vi "initialize_driver_session.vi"(4 "Supported instruments":string[](array[string]), 5 "Repeated Capabilities":T4[](array[typedef]), 6 "Attributes":T2[](array[typedef]) {"Flags" format="%08b"; "Access" items=["Read Only", "Write Only", "Read/Write"]; "Data Type" items=["Integer 32", "Double", "String", "Boolean", "None", "Integer 64", "RawString"]}, 7 "Range Tables":T3[](array[typedef]) {"Type" items=["Range", "Coerced", "Discrete"]}, 8 "error in":errorcluster caption="error in (no error)", 9 "Option String":string, 10 "Non-VXI sessions list (\"ASRL,SOCKET\")":T1[](array[typedef])=[enum."ASRL", enum."SOCKET"], 11 "VISA resource name":refnum<visa-resource-name>) -> (0 "error out":errorcluster, 2 "Simulation *IDN? response out":string, 3 "VISA resource name out":refnum<visa-resource-name>)   [LabVIEW 2022 SP3, in "hmp4000_rsidr_core.lvlib"]
uses:
  hmp4000_rsidr_core.lvlib
  type_Input_Format_RepCap.ctl
  type_Input_Format_RangeTable.ctl
  type_Input_Format_Attribute.ctl
  type_InterfaceType.ctl
  type_Error_Codes.ctl
  type_Session_Parameter_int32.ctl
  type_Session_Data.ctl
  type_VisaAccessMode.ctl
  type_OPC_Wait_Mode.ctl
  type_Binary_Float_Number_Format.ctl
  type_Binary_Integer_Number_Format.ctl
  _type_Operation_Fgv_Attributes.ctl
  _type_Operation_Fgv_Cache.ctl
  _type_Operation_Fgv_RangeTable.ctl
  type_AdditionalFlag_Bits.ctl
  _type_Operation_Fgv_Session.ctl
  type_Session_Parameter_Boolean.ctl
  Trim Whitespace One-Sided.vi
  Match Regular Expression.xnode
  _type_Operation_Fgv_Debug.ctl
panel:
  # "Attribute Flags:\nbit 0: OPC Wait\nbit 1: No Status Check\nbit 2: Cache only\nbit 3: Hidden"
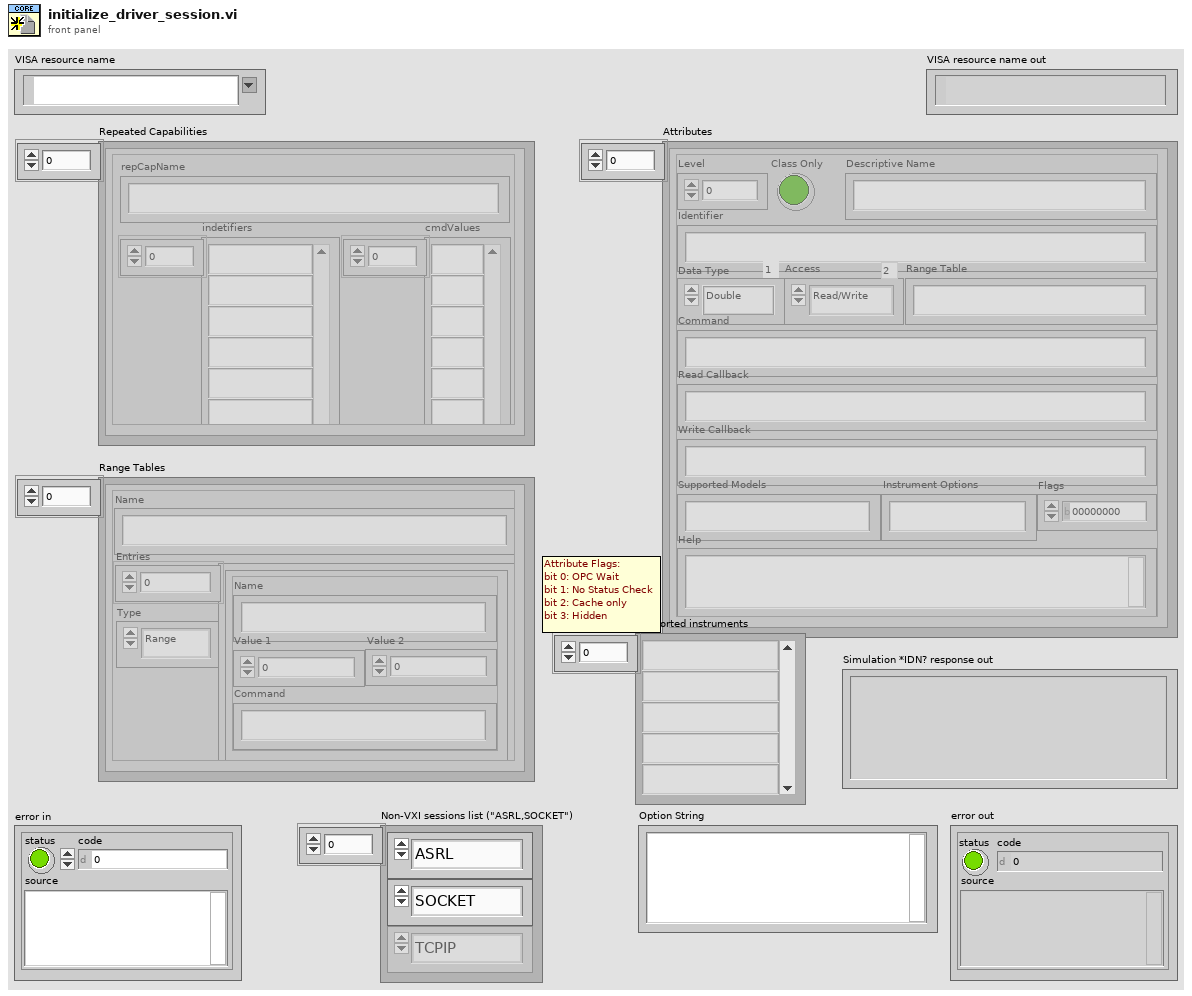
[diagram p1: front panel]
types:
  T1 = typedef "hmp4000_rsidr_core.lvlib/type_InterfaceType.ctl" = enum16{"Unknown", "GPIB", "VXI", "GPIB_VXI", "ASRL", "PXI", "TCPIP", "USB", "SOCKET"}
  T2 = typedef "hmp4000_rsidr_core.lvlib/type_Input_Format_Attribute.ctl" = cluster{"Level":i32, "Class Only":bool, "Identifier":string, "Descriptive Name":string, "Data Type":u16, "Command":string, "Access":u16, "Range Table":string, "Read Callback":string, "Write Callback":string, "Supported Models":string, "Instrument Options":string, "Flags":i32, "Help":string}
  T3 = typedef "hmp4000_rsidr_core.lvlib/type_Input_Format_RangeTable.ctl" = cluster{"Type":u16, "Name":string, "Entries":cluster{"Name":string, "Value 1":dbl, "Value 2":dbl, "Command":string}[]}
  T4 = typedef "hmp4000_rsidr_core.lvlib/type_Input_Format_RepCap.ctl" = cluster{"repCapName":string, "indetifiers":string[], "cmdValues":string[]}
  T5 = typedef "hmp4000_rsidr_core.lvlib/_type_Operation_Fgv_RangeTable.ctl" = enum16{"Initialize", "Check", "Coerce", "Get Command String", "Get Numeric Value", "Get Default Value", "Get Range Table Type"}
  T6 = typedef "hmp4000_rsidr_core.lvlib/_type_Operation_Fgv_Cache.ctl" = enum16{"Initialize", "Get Cached Value", "Set Cached Value", "Clear"}
  T7 = typedef "hmp4000_rsidr_core.lvlib/_type_Operation_Fgv_Attributes.ctl" = enum16{"Initialize", "Get Attribute"}
  T8 = typedef "hmp4000_rsidr_core.lvlib/type_Session_Data.ctl" = cluster{"IDN string":string, "Instrument FW":string, "Instr type":string, "Instr type for err. msg.":string, "Installed Options":string[], "Ignore Error Messages":string, "Logging params":variant, "OPC Timeout":i32, "VISA Timeout":i32, "STB Poll VISA Timeout":i32, "Additional Flags":i32, "Wait Before Read":i32, "Wait Before Write":i32, "Option String Flags":i32, "IO Segment Size":i64, "VISA Access Mode":T9, "Interface Type":T1, "OPC Wait Mode":T10, "Bin Float Number  Format":T11, "Bin Integer Number Format":T12, "Simulate":bool, "VXIcapable":bool, "Duplicate Session":bool, "Add LF to Write":bool, "Logging":bool, "Fast Sweep":bool, "Query Instrument Status":bool, "Check Range":bool, "Check Options":bool}
  T9 = typedef "hmp4000_rsidr_core.lvlib/type_VisaAccessMode.ctl" = u16
  T10 = typedef "hmp4000_rsidr_core.lvlib/type_OPC_Wait_Mode.ctl" = enum16{"STBpolling", "STBpollingSlow", "STBpollingSuperSlow", "ServiceRequest", "OPCquery"}
  T11 = typedef "hmp4000_rsidr_core.lvlib/type_Binary_Float_Number_Format.ctl" = enum16{"Float_4_Bytes_Swapped", "Float_4_Bytes", "Double_8_Bytes_Swapped", "Double_8_Bytes"}
  T12 = typedef "hmp4000_rsidr_core.lvlib/type_Binary_Integer_Number_Format.ctl" = enum16{"Int32_4_Bytes_Swapped", "Int32_4 Bytes", "Int16_2_Bytes_Swapped", "Int16_2_Bytes"}
  T13 = typedef "hmp4000_rsidr_core.lvlib/type_Session_Parameter_int32.ctl" = enum16{"OPC Timeout", "Additional Flags", "Wait Before Write", "Wait Before Read", "Bin Data Chunk Size", "VISA Access Mode", "VISA Timeout", "Bin Float Number Format", "Bin Integer Number Format", "STBpollVISAtimeout", "OPCwaitMode"}
  T14 = typedef "hmp4000_rsidr_core.lvlib/type_Error_Codes.ctl" = enum16{"No_error", "VISA_err_ResourceNotFound", "VISA_err_Timeout", "VISA_warn_MoreDataAvailable", "RS_err_MissingCallback", "RS_err_InvalidAttribute", "RS_err_InvalidValue", "RS_err_UnknownResource", "RS_err_AlreadyInitialized", "RS_err_InstrumentStatus", "RS_err_BadRepCapName", "RS_err_TypesMismatch", "RS_err_ValueNotSupported", "RS_err_InvalidRngTable", "RS_err_IDqueryFail", "RS_err_UnexpResponse", "VISA_warn_ConfigNotLoaded", "RS_err_AttributeNotReadable", "RS_err_AttributeNotWritable", "RS_err_InstrumentType", "RS_err_InstrumentOption", "VISA_err_InvalidSize", "RS_err_ReliabilityIndicator", "VISA_warn_UnknownStatus", "VISA_warn_TermCharRead", "VISA_err_IO_error", "RS_err_FunctionNotSupported", "VISA_warn_QueueEmpty"}
  T15 = typedef "hmp4000_rsidr_core.lvlib/type_AdditionalFlag_Bits.ctl" = enum16{"Send LF after Bin Block", "Junk read with io_clear_buffers.vi", "io_clear_buffers: viClear()", "io_clear_buffers: viFlush()", "<NotUsed1>", "Allow Dbl & Int Bin/Ascii read", "*OPC? in check_instrument_error.vi", "<NotUsed2>", "Smart Enum Matching", "Less Strict RepCaps check", "AssureResponseEndWithLF"}
  T16 = typedef "hmp4000_rsidr_core.lvlib/_type_Operation_Fgv_Session.ctl" = enum16{"Initialize", "GetData", "SetData", "Clear", "GetSessionIx"}
  T17 = typedef "hmp4000_rsidr_core.lvlib/type_Session_Parameter_Boolean.ctl" = enum16{"Simulate", "Query Instr Status", "Check Range", "Check Options", "Add LF to Write", "Duplicate Session", "Fast Sweep", "Logging"}
  T18 = enum16{"Unknown", "GPIB", "VXI", "GPIB_VXI", "ASRL", "PXI", "TCPIP", "USB", "SOCKET"}
  T19 = typedef "hmp4000_rsidr_core.lvlib/_type_Operation_Fgv_Debug.ctl" = enum16{"Reset", "ReadCommand", "SetCommand"}
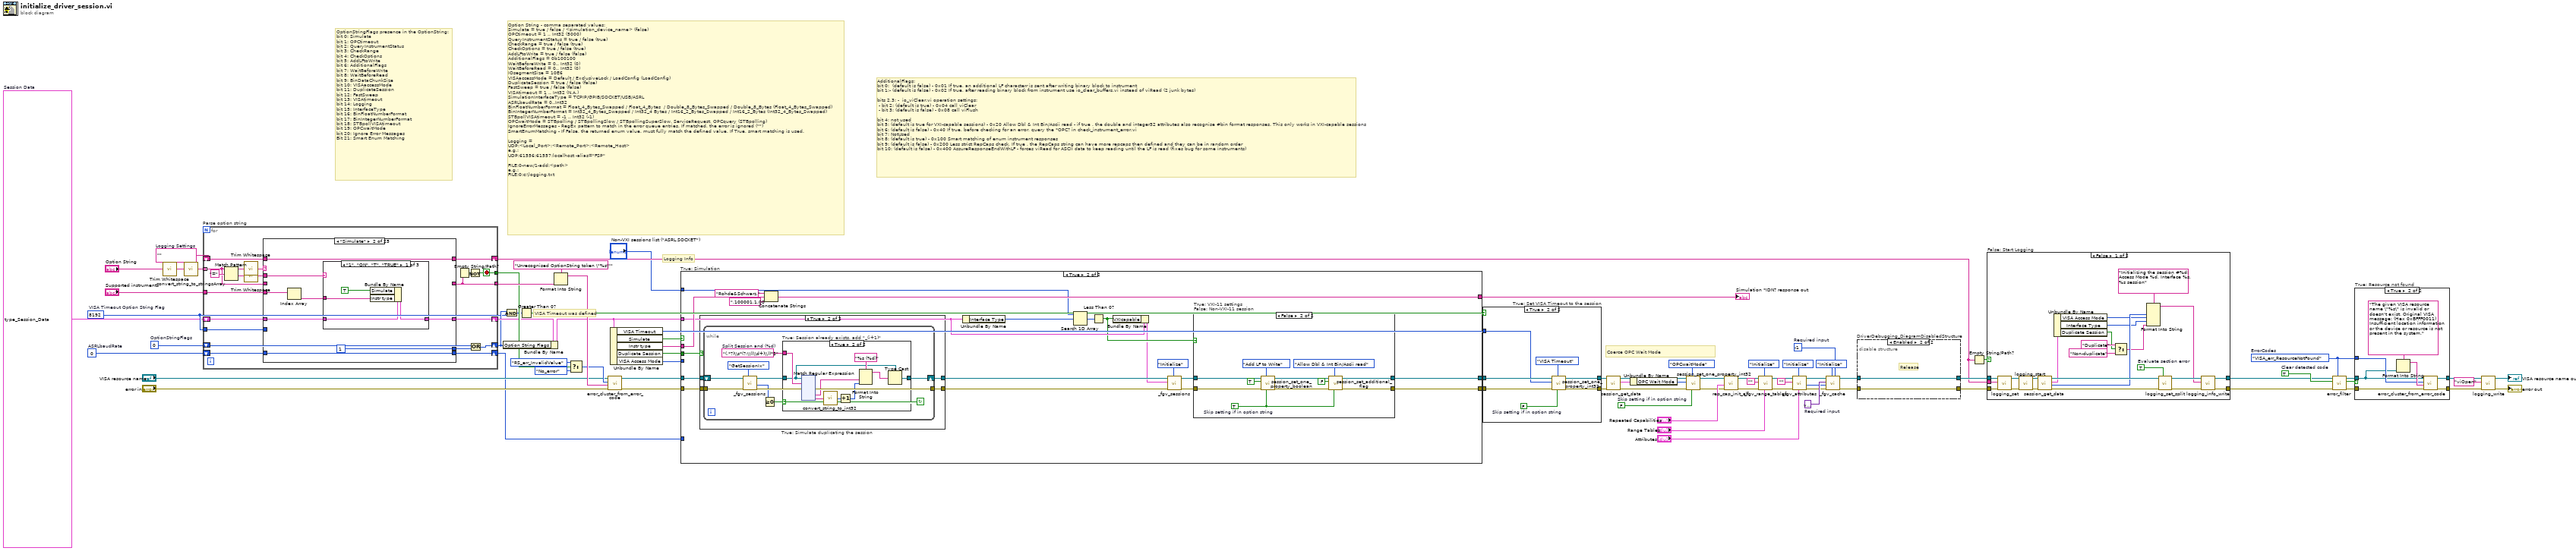
[diagram p0: block diagram]
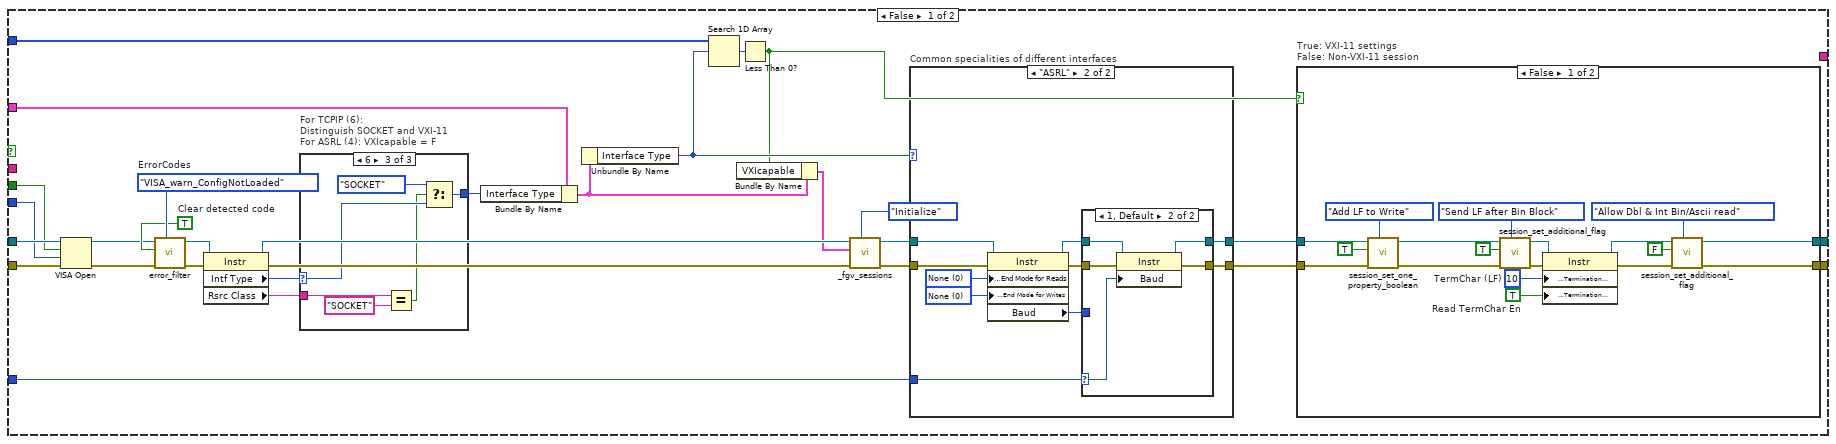
[diagram p3: hidden frame]
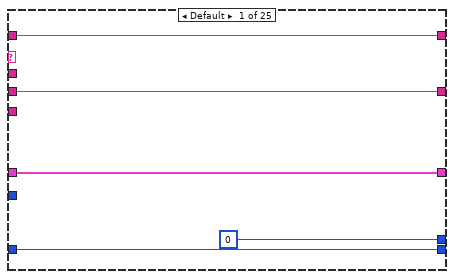
[diagram p14: hidden frame]
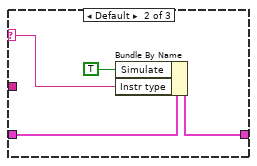
[diagram p15: hidden frame]
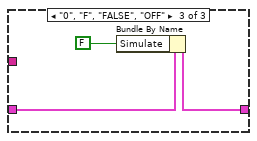
[diagram p16: hidden frame]
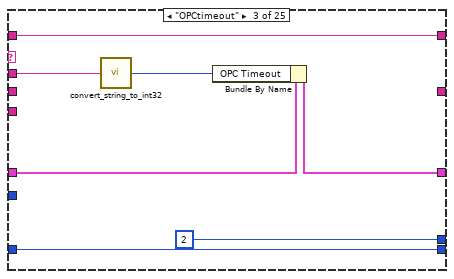
[diagram p17: hidden frame]
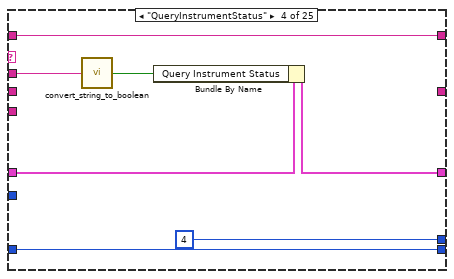
[diagram p18: hidden frame]
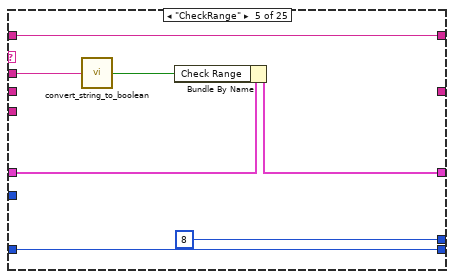
[diagram p19: hidden frame]
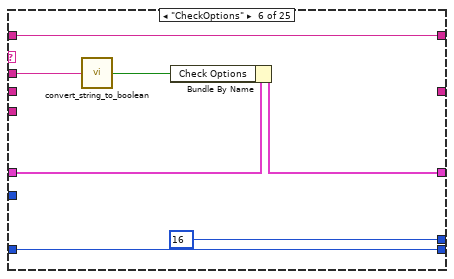
[diagram p20: hidden frame]
diagram:
  w4 = T8 {"IDN string"="", "Instrument FW"="", "Instr type"="", "Instr type for err. msg."="", "Installed Options"=[], "Ignore Error Messages"="", "Logging params"=variant, "OPC Timeout"=10000, "VISA Timeout"=5000, "STB Poll VISA Timeout"=-1, "Additional Flags"=292, "Wait Before Read"=0, "Wait Before Write"=0, "Option String Flags"=0, "IO Segment Size"=10000000, "VISA Access Mode"=4, "Interface Type"=enum."Unknown", "OPC Wait Mode"=enum."STBpolling", "Bin Float Number  Format"=enum."Float_4_Bytes_Swapped", "Bin Integer Number Format"=enum."Int32_4_Bytes_Swapped", "Simulate"=FALSE, "VXIcapable"=FALSE, "Duplicate Session"=FALSE, "Add LF to Write"=FALSE, "Logging"=FALSE, "Fast Sweep"=FALSE, "Query Instrument Status"=TRUE, "Check Range"=TRUE, "Check Options"=TRUE}  # Session Data
  w7 = FALSE  # Skip setting if in option string
  w18 = 0  # ASRLbaudRate
  w31 = 8192  # VISA Timeout Option String Flag
  w37 = 0  # OptionStringFlags
  w57 = type_Error_Codes."VISA_err_ResourceNotFound"  # ErrorCodes
  w59 = TRUE  # Clear detected code
  w66 = ""  # Logging Settings
  w80 = variant  # Required input
  w38 = -1  # Required input
  # "Coerce OPC Wait Mode"
  # "VISA Timeout was defined"
  # "Logging Info"
  # "OptionStringFlags presence in the OptionString:\nbit 0: Simulate\nbit 1: OPCtimeout\nbit 2: QueryInstrumentStatus\nbit 3: CheckRange\nbit 4: CheckOptions\nbit 5: AddLFtoWrite\nbit 6: AdditionalFlags\nbit 7: WaitBeforeWrite\nbit 8: WaitBeforeRead\nbit 9: BinDataChunkSize\nbit 10: VISAaccessMode\nbit 11: DuplicateSession\nbit 12: FastSweep\nbit 13: VISAtimeout\nbit 14: Logging\nbit 15: InterfaceType\nbit 16: BinFloatNumberFormat\nbit 17: BinIntegerNumberFormat\nbit 18: STBpollVISAtimeout\nbit 19: OPCwaitMode\nbit 20: Ignore Error Messages\nBit 21: Smart Enum Matching"
  # "AdditionalFlags:\nbit 0:  (default is false) - 0x01 If true, an additional LF characterr is sent after writing binary block to instrument\nbit 1:- (default is false) - 0x02 If true, after reading binary block from instrument use io_clear_buffers.vi instead of viRead (2 junk bytes)\n\nbits 2,3: -  io_viClear.vi operation settings:\n - bit 2: (default is true) - 0x04 call viClear\n - bit 3: (default is false) - 0x08 call viFlush\n\nbit 4: not used\nbit 5: (default is true for VXI-capable sessions) - 0x20 Allow Dbl & Int Bin/Ascii read - if true , the double and integer32 attributes also recognise #bin format responses. This only works in VXI-capable sessions\nbit 6: (default is false) - 0x40 If true, before checking for an error, query the *OPC? in check_instrument_error.vi\nbit 7: NotUsed\nbit 8: (default is true) - 0x100 Smart matching of enum instrument responses\nbit 9: (default is false) - 0x200 Less strict RepCaps check. If true , the RepCaps string can have more repcaps then defined and they can be in random order\nbit 10: (default is false) - 0x400 AssureResponseEndWithLF - forces viRead for ASCII data to keep reading until the LF is read (fixes bug for some instruments)"
  # "Option String - comma separated values:\nSimulate = true / false / <simulation_device_name> (false)\nOPCtimeout = 1 .. Int32 (5000)\nQueryInstrumentStatus = true / false (true)\nCheckRange = true / false (true)\nCheckOptions = true / false (true)\nAddLFtoWrite = true / false (false)\nAdditionalFlags = 0b100100\nWaitBeforeWrite = 0.. Int32 (0)\nWaitBeforeRead = 0.. Int32 (0)\nIOsegmentSize = 10E6\nVISAaccessMode = Default / ExclusiveLock / LoadConfig (LoadConfig)\nDuplicateSession = true / false (false)\nFastSweep = true / false (false)\nVISAtimeout = 1 .. Int32 (N.A.)\nSimulationInterfaceType = TCPIP/GPIB/SOCKET/USB/ASRL\nASRLbaudRate = 0..Int32\nBinFloatNumberFormat = Float_4_Bytes_Swapped / Float_4_Bytes  / Double_8_Bytes_Swapped / Double_8_Bytes (Float_4_Bytes_Swapped)\nBinIntegerNumberFormat = Int32_4_Bytes_Swapped / Int32_4 Bytes / Int16_2_Bytes_Swapped / Int16_2_Bytes (Int32_4_Bytes_Swapped)\nSTBpollVISAtimeout = -1 .. Int32 (-1)\nOPCwaitMode = STBpolling / STBpollingSlow / STBpollingSuperSlow, ServiceRequest, OPCquery (STBpolling)\nIgnoreErrorMessages - RegEx pattern to match in the error queue entries. If matched, the error is ignored (\"\")\nSmartEnumMatching - If False, the returned enum value. must fully match the defined value. If True, smart matching is used.\n\nLogging =\nUDP:<Local_Port>:<Remote_Port>:<Remote_Host>\ne.g.:\nUDP:61556:61557:localhost -alias=\"FSP\"\n\nFILE:0-new/1-add:<path>\ne.g.:\nFILE:0:c:\\logging.txt"
  n1 = call "Trim Whitespace.vi"("string"="Option String") -> ("trimmed string"=w6:string)  [unwired: 1 in]
  n2 = call "convert_string_to_stringsArray.vi"("String in"=w6) -> ("string array out"=w70:string[])  [unwired: 3 in, 1 out]
  n3 = for "Parse option string" {
    tunnel: w70 -> [w94] mode=indexing
    shift-right: [w96] -> w33
    shift-left: w4 -> [w97]
    tunnel: "Supported instruments" -> [w92]
    shift-right: [w90] -> w64
    shift-left: w66 -> [w91]
    tunnel: [w88] -> w44
    tunnel: [w87] -> w43
    shift-right: [w85] -> w32
    shift-left: w37 -> [w86]
    tunnel: w31 -> [w83]
    shift-right: [w81] -> w17
    shift-left: w18 -> [w82]
    stop <- w87 stop-if-true
    n4 = Match Pattern(string=w94, regular expression="=") -> (before substring=w99:string, after substring=w98:string)  [unwired: 1 in, 2 out]
    n5 = call "Trim Whitespace.vi"("string"=w99) -> ("trimmed string"=w95:string)  [unwired: 1 in]
    n6 = call "Trim Whitespace.vi"("string"=w98) -> ("trimmed string"=w93:string)  [unwired: 1 in]
    n7 = case shown="\"Simulate\"" w95 {
      tunnel: w97 -> [w105 w107 w131 w133 w140 w152 w154 w166 w173 w183 w190 w198 w200 w214 w221 w228 w235 w241 w244 w260 w275 w291 w297 w314 w324]
      tunnel: [w105 w106 w130 w132 w139 w146 w153 w165 w174 w182 w189 w197 w199 w213 w220 w227 w235 w241 w243 w259 w274 w290 w296 w313 w325] -> w96
      tunnel: w94 -> [w103 _ _ _ _ _ _ _ _ _ _ _ w205 _ _ _ _ _ w249 w265 w280 _ w302 _ _]
      tunnel: w93 -> [_ w109 w128 w137 w144 w150 w158 w163 w170 w180 w187 w195 w207 w218 w225 w232 w237 w242 w251 w267 w282 w293 w304 w312 w321]
      tunnel: w92 -> [_ w113 _ _ _ _ _ _ _ _ _ _ _ _ _ _ _ _ _ _ _ _ _ _ _]
      tunnel: w91 -> [w104 w112 w129 w138 w145 w151 w159 w164 w176 w181 w188 w196 w206 w219 w226 w233 w238 _ w250 w266 w281 w289 w303 w317 w327]
      tunnel: [w104 w112 w129 w138 w145 w151 w159 w164 w176 w181 w188 w196 w206 w219 w226 w233 w238 w242 w250 w266 w281 w289 w303 w317 w327] -> w90
      tunnel: [w103 _ _ _ _ _ _ _ _ _ _ _ w204 _ _ _ _ _ w248 w264 w279 _ w301 _ _] -> w88
      tunnel: [0 ("y") 1 ("y") 2 ("y") 4 ("y") 8 ("y") 16 ("y") 32 ("y") 64 ("y") 64 ("y") 128 ("y") 256 ("y") 512 ("y") 1024 ("y") 2048 ("y") 4096 ("y") w230 w234 16384 ("y") 32768 ("y") 65536 ("y") 131072 ("y") 262144 ("y") 524288 ("y") 1048576 ("y") 64 ("y")] -> w84
      tunnel: w83 -> [_ _ _ _ _ _ _ _ _ _ _ _ _ _ _ w230 _ _ _ _ _ _ _ _ _]
      tunnel: w82 -> [w101 w110 w125 w134 w141 w147 w155 w160 w175 w177 w184 w192 w201 w215 w222 w229 _ w239 w245 w261 w276 w294 w298 w315 w326]
      tunnel: [w101 w110 w125 w134 w141 w147 w155 w160 w175 w177 w184 w192 w201 w215 w222 w229 w236 w239 w245 w261 w276 w294 w298 w315 w326] -> w81
      frame Default {
      }
      frame "Simulate" {
        n8 = Index Array(array=w113) -> (element=w108:string)  [unwired: 1 in]
        n9 = case shown="\"1\", \"ON\", \"T\", \"TRUE\"" w109 {
          selector: w109 -> [_ w118 _]
          tunnel: w107 -> [w117 w121 w124]
          tunnel: [w116 w120 w123] -> w106
          tunnel: w108 -> [w115 _ _]
          frame "1", "ON", "T", "TRUE" {
            n10 = Bundle By Name(cluster=w117, "Simulate"=TRUE ("Simulation"), "Instr type"=w115) -> (w116:T8)
          }
          frame Default {
            n11 = Bundle By Name(cluster=w121, "Simulate"=TRUE ("Simulation"), "Instr type"=w118) -> (w120:T8)
          }
          frame "0", "F", "FALSE", "OFF" {
            n12 = Bundle By Name(cluster=w124, "Simulate"=FALSE ("Simulation")) -> (w123:T8)
          }
        }
      }
      frame "OPCtimeout" {
        n13 = call "convert_string_to_int32.vi"("String in"=w128) -> ("int32 value out"=w127:i32)  [unwired: 4 in]
        n14 = Bundle By Name(cluster=w131, "OPC Timeout"=w127) -> (w130:T8)
      }
      frame "QueryInstrumentStatus" {
        n15 = call "convert_string_to_boolean.vi"("String in"=w137) -> ("boolean value out"=w136:bool)  [unwired: 4 in]
        n16 = Bundle By Name(cluster=w133, "Query Instrument Status"=w136) -> (w132:T8)
      }
      frame "CheckRange" {
        n17 = call "convert_string_to_boolean.vi"("String in"=w144) -> ("boolean value out"=w143:bool)  [unwired: 4 in]
        n18 = Bundle By Name(cluster=w140, "Check Range"=w143) -> (w139:T8)
      }
      frame "CheckOptions" {
        n19 = call "convert_string_to_boolean.vi"("String in"=w150) -> ("boolean value out"=w149:bool)  [unwired: 4 in]
        n20 = Bundle By Name(cluster=w152, "Check Options"=w149) -> (w146:T8)
      }
      frame "AddLFtoWrite" {
        n21 = call "convert_string_to_boolean.vi"("String in"=w158) -> ("boolean value out"=w157:bool)  [unwired: 4 in]
        n22 = Bundle By Name(cluster=w154, "Add LF to Write"=w157) -> (w153:T8)
      }
      frame "AdditionalFlags" {
        n23 = call "convert_string_to_int32.vi"("String in"=w163) -> ("int32 value out"=w162:i32)  [unwired: 4 in]
        n24 = Bundle By Name(cluster=w166, "Additional Flags"=w162) -> (w165:T8)
      }
      frame "AssureResponseEndWithLF" {
        n25 = Unbundle By Name(w173) -> ("Additional Flags"=w172:i32)
        n26 = call "convert_string_to_boolean.vi"("String in"=w170) -> ("boolean value out"=w169:bool)  [unwired: 4 in]
        n27 = call "_session_set_additionalFlag_value.vi"("New value in"=w169, "AdditionalFlag bit"=type_AdditionalFlag_Bits."AssureResponseEndWithLF", "Additional Flags in"=w172) -> ("Additional Flags out"=w168:i32)  [unwired: 1 in, 1 out]
        n28 = Bundle By Name(cluster=w173, "Additional Flags"=w168) -> (w174:T8)
      }
      frame "WaitBeforeWrite" {
        n29 = call "convert_string_to_int32.vi"("String in"=w180) -> ("int32 value out"=w179:i32)  [unwired: 4 in]
        n30 = Bundle By Name(cluster=w183, "Wait Before Write"=w179) -> (w182:T8)
      }
      frame "WaitBeforeRead" {
        n31 = call "convert_string_to_int32.vi"("String in"=w187) -> ("int32 value out"=w186:i32)  [unwired: 4 in]
        n32 = Bundle By Name(cluster=w190, "Wait Before Read"=w186) -> (w189:T8)
      }
      frame "IOsegmentSize" {
        n33 = call "convert_string_to_int32.vi"("String in"=w195) -> ("int32 value out"=w194:i32)  [unwired: 4 in]
        n34 = To Quad Integer(1:w194) -> (0:w191:i64)
        n35 = Bundle By Name(cluster=w198, "IO Segment Size"=w191) -> (w197:T8)
      }
      frame "VISAaccessMode" {
        n36 = case shown="\"LoadConfig\"" w207 {
          tunnel: w205 -> [_ w210 _ _]
          tunnel: [_ w210 _ _] -> w204
          tunnel: [w208 w209 w211 w212] -> w203
          frame "Default" {
            w208 = T9 0 items=["VISA Defaults"=0, "Exclusive Lock"=1, "Load Settings"=4]  # VISA Access Mode
          }
          frame Default {
            w209 = T9 4 items=["VISA Defaults"=0, "Exclusive Lock"=1, "Load Settings"=4]  # VISA Access Mode
          }
          frame "ExclusiveLock" {
            w211 = T9 1 items=["VISA Defaults"=0, "Exclusive Lock"=1, "Load Settings"=4]  # VISA Access Mode
          }
          frame "LoadConfig" {
            w212 = T9 4 items=["VISA Defaults"=0, "Exclusive Lock"=1, "Load Settings"=4]  # VISA Access Mode
          }
        }
        n37 = Bundle By Name(cluster=w200, "VISA Access Mode"=w203) -> (w199:T8)
      }
      frame "DuplicateSession" {
        n38 = call "convert_string_to_boolean.vi"("String in"=w218) -> ("boolean value out"=w217:bool)  [unwired: 4 in]
        n39 = Bundle By Name(cluster=w214, "Duplicate Session"=w217) -> (w213:T8)
      }
      frame "FastSweep" {
        n40 = call "convert_string_to_boolean.vi"("String in"=w225) -> ("boolean value out"=w224:bool)  [unwired: 4 in]
        n41 = Bundle By Name(cluster=w221, "Fast Sweep"=w224) -> (w220:T8)
      }
      frame "VISAtimeout" {
        n42 = call "convert_string_to_int32.vi"("String in"=w232) -> ("int32 value out"=w231:i32)  [unwired: 4 in]
        n43 = Bundle By Name(cluster=w228, "VISA Timeout"=w231) -> (w227:T8)
      }
      frame "ASRLbaudRate" {
        w234 = 0  # OptionStringFlags
        n44 = call "convert_string_to_int32.vi"("String in"=w237) -> ("int32 value out"=w236:i32)  [unwired: 4 in]
      }
      frame "Logging" {
      }
      frame "SimulationInterfaceType" {
        n45 = case shown="\"ASRL\"" w251 {
          tunnel: w249 -> [w253 _ _ _ _ _]
          tunnel: [w253 _ _ _ _ _] -> w248
          tunnel: [type_InterfaceType."TCPIP" ("Interface Type") type_InterfaceType."TCPIP" ("Interface Type") type_InterfaceType."GPIB" ("Interface Type") type_InterfaceType."SOCKET" ("Interface Type") type_InterfaceType."USB" ("Interface Type") type_InterfaceType."ASRL" ("Interface Type")] -> w247
          frame Default {
          }
          frame "TCPIP" {
          }
          frame "GPIB" {
          }
          frame "SOCKET" {
          }
          frame "USB" {
          }
          frame "ASRL" {
          }
        }
        n46 = Bundle By Name(cluster=w244, "Interface Type"=w247) -> (w243:T8)
      }
      frame "BinFloatNumberFormat" {
        n47 = case shown="\"Double_8_Bytes_Swapped\"" w267 {
          tunnel: w265 -> [w269 _ _ _ _]
          tunnel: [w269 _ _ _ _] -> w264
          tunnel: [w268 w270 w271 w272 w273] -> w263
          frame Default {
            w268 = type_Binary_Float_Number_Format."Float_4_Bytes_Swapped"  # Bin Number Format
          }
          frame "Float_4_Bytes_Swapped" {
            w270 = type_Binary_Float_Number_Format."Float_4_Bytes_Swapped"  # Bin Float Number Format
          }
          frame "Float_4_Bytes" {
            w271 = type_Binary_Float_Number_Format."Float_4_Bytes"  # Bin Float Number Format
          }
          frame "Double_8_Bytes_Swapped" {
            w272 = type_Binary_Float_Number_Format."Double_8_Bytes_Swapped"  # Bin Float Number Format
          }
          frame "Double_8_Bytes" {
            w273 = type_Binary_Float_Number_Format."Double_8_Bytes"  # Bin Float Number Format
          }
        }
        n48 = Bundle By Name(cluster=w260, "Bin Float Number  Format"=w263) -> (w259:T8)
      }
      frame "BinIntegerNumberFormat" {
        n49 = case shown="\"Int16_2_Bytes_Swapped\"" w282 {
          tunnel: w280 -> [w284 _ _ _ _]
          tunnel: [w284 _ _ _ _] -> w279
          tunnel: [w283 w285 w286 w287 w288] -> w278
          frame Default {
            w283 = type_Binary_Integer_Number_Format."Int32_4_Bytes_Swapped"  # Bin Integer Number Format
          }
          frame "Int32_4_Bytes_Swapped" {
            w285 = type_Binary_Integer_Number_Format."Int32_4_Bytes_Swapped"  # Bin Integer Number Format
          }
          frame "Int32_4_Bytes" {
            w286 = type_Binary_Integer_Number_Format."Int32_4 Bytes"  # Bin Integer Number Format
          }
          frame "Int16_2_Bytes_Swapped" {
            w287 = type_Binary_Integer_Number_Format."Int16_2_Bytes_Swapped"  # Bin Integer Number Format
          }
          frame "Int16_2_Bytes" {
            w288 = type_Binary_Integer_Number_Format."Int16_2_Bytes"  # Bin Integer Number Format
          }
        }
        n50 = Bundle By Name(cluster=w275, "Bin Integer Number Format"=w278) -> (w274:T8)
      }
      frame "STBpollVISAtimeout" {
        n51 = call "convert_string_to_int32.vi"("String in"=w293) -> ("int32 value out"=w292:i32)  [unwired: 4 in]
        n52 = Bundle By Name(cluster=w291, "STB Poll VISA Timeout"=w292) -> (w290:T8)
      }
      frame "OPCwaitMode" {
        n53 = case shown="\"ServiceRequest\"" w304 {
          tunnel: w302 -> [_ _ _ _ _ w310]
          tunnel: [_ _ _ _ _ w310] -> w301
          tunnel: [w305 w306 w307 w308 w309 w311] -> w300
          frame "STBpolling" {
            w305 = type_OPC_Wait_Mode."STBpolling"  # OPC Wait Mode
          }
          frame "STBpollingSlow" {
            w306 = type_OPC_Wait_Mode."STBpollingSlow"  # OPC Wait Mode
          }
          frame "STBpollingSuperSlow" {
            w307 = type_OPC_Wait_Mode."STBpollingSuperSlow"  # OPC Wait Mode
          }
          frame "ServiceRequest" {
            w308 = type_OPC_Wait_Mode."ServiceRequest"  # OPC Wait Mode
          }
          frame "OPCquery" {
            w309 = type_OPC_Wait_Mode."OPCquery"  # OPC Wait Mode
          }
          frame Default {
            w311 = type_OPC_Wait_Mode."STBpolling"  # OPC Wait Mode
          }
        }
        n54 = Bundle By Name(cluster=w297, "OPC Wait Mode"=w300) -> (w296:T8)
      }
      frame "IgnoreErrorMessages" {
        n55 = Bundle By Name(cluster=w314, "Ignore Error Messages"=w312) -> (w313:T8)
      }
      frame "SmartEnumMatching" {
        n56 = Unbundle By Name(w324) -> ("Additional Flags"=w323:i32)
        n57 = call "convert_string_to_boolean.vi"("String in"=w321) -> ("boolean value out"=w320:bool)  [unwired: 4 in]
        n58 = call "_session_set_additionalFlag_value.vi"("New value in"=w320, "AdditionalFlag bit"=type_AdditionalFlag_Bits."Smart Enum Matching", "Additional Flags in"=w323) -> ("Additional Flags out"=w319:i32)  [unwired: 1 in, 1 out]
        n59 = Bundle By Name(cluster=w324, "Additional Flags"=w319) -> (w325:T8)
      }
    }
    n60 = Empty String/Path?(string/path=w88) -> (empty?=w89:bool)
    n61 = Not(x=w89) -> (.not. x?=w87:bool)
    n62 = Or(x=w86, y=w84) -> (x .or. y?=w85:i32)
  }
  n63 = Bundle By Name(cluster=w33, "Option String Flags"=w32) -> (w36:T8)
  n64 = And(x=w32, y=w31) -> (x .and. y?=w30:i32)
  n65 = Greater Than 0?(x=w30) -> (x > 0?=w29:bool)
  n66 = Format Into String(format string="Unrecognised OptionString token \"%s\"", w44) -> (resulting string=w46:string)  [unwired: 2 in, 1 out]
  n67 = Select(t=type_Error_Codes."RS_err_InvalidValue" ("Error Enum in"), s=w43, f=type_Error_Codes."No_error" ("Error Enum in")) -> (s? t:f=w40:T14)
  n68 = call "error_cluster_from_error_code.vi"("error in"="error in", "Error Message (\"\")"=w46, "Error Enum in"=w40, "VISA resource name"="VISA resource name") -> ("error out"=w25:errorcluster, "VISA resource name out"=w24:refnum<visa-resource-name>)  [unwired: 6 in]
  n69 = Unbundle By Name(w36) -> ("VISA Timeout"=w28:i32, "Simulate"=w56:bool, "Instr type"=w58:string, "Duplicate Session"=w23:bool, "VISA Access Mode"=w22:T9)
  n70 = case "True: Simulation" shown="True" w56 {
    tunnel: w24 -> [w356 w421]
    tunnel: w25 -> [w357 w420]
    tunnel: [w336 w414] -> w35
    tunnel: [w335 w413] -> w34
    tunnel: w58 -> [_ w419]
    tunnel: [_ w423] -> w55
    tunnel: w36 -> [w346 w412]
    tunnel: w23 -> [w349 w422]
    tunnel: w22 -> [w348 _]
    tunnel: w17 -> [w339 _]
    tunnel: "Non-VXI sessions list (\"ASRL,SOCKET\")" -> [w333 w410]
    frame False {
      w350 = TRUE  # Clear detected code
      w353 = type_Error_Codes."VISA_warn_ConfigNotLoaded"  # ErrorCodes
      n71 = VISA Open ("Open instrument")(duplicate session (F)=w349, access mode=w348, error in (no error)=w357, VISA resource name=w356) -> (VISA resource name=w345:refnum<visa-resource-name>, error out=w344:errorcluster)  [unwired: 1 in]
      n72 = call "error_filter.vi"("Error Enum in"=w353, "error in"=w344, "Clear detected code (F)"=w350, "VISA resource name"=w345) -> ("error out"=w352:errorcluster, "VISA resource name out"=w351:refnum<visa-resource-name>)  [unwired: 5 in, 1 out]
      n73 = property on="Property Node" class="Instr"(reference=w351, error in=w352) -> (reference out=w342:refnum<visa-resource-name>, error out=w343:errorcluster, "Intf Type"=w355:u16, "Rsrc Class"=w354:string)
      n74 = case "For TCPIP (6):\nDistinguish SOCKET and VXI-11\nFor ASRL (4): VXIcapable = F" shown="6" w355 {
        selector: w355 -> [w397 w398 w402]
        tunnel: w354 -> [_ _ w404]
        tunnel: [w397 w398 w401] -> w347
        frame Default {
        }
        frame 4 {
        }
        frame 6 {
          n75 = Equal?(x=w404, y="SOCKET") -> (x = y?=w399:bool)
          n76 = Select(t=T18."SOCKET" ("Interface Type"), s=w399, f=w402) -> (s? t:f=w401:u16)
        }
      }
      n77 = Bundle By Name(cluster=w346, "Interface Type"=w347) -> (w330:T8)
      n78 = Unbundle By Name(w330) -> ("Interface Type"=w332:T1)
      n79 = Search 1D Array(1D array=w333, element=w332) -> (index of element=w334:i32)  [unwired: 1 in]
      n80 = Less Than 0?(x=w334) -> (x < 0?=w329:bool)
      n81 = Bundle By Name(cluster=w330, "VXIcapable"=w329) -> (w331:T8)
      n82 = call "_fgv_sessions.vi"("Operation"=_type_Operation_Fgv_Session."Initialize", "error in"=w343, "Session User Data in (None)"=w331, "VISA resource name"=w342) -> ("error out"=w341:errorcluster, "VISA resource name out"=w340:refnum<visa-resource-name>)  [unwired: 4 in, 2 out]
      n83 = case "Common specialities of different interfaces" shown="\"ASRL\"" w332 {
        tunnel: w341 -> [w378 w382]
        tunnel: w340 -> [w379 w381]
        tunnel: [w378 w384] -> w338
        tunnel: [w379 w383] -> w337
        tunnel: w339 -> [_ w387]
        frame Default {
        }
        frame "ASRL" {
          w388 = u16 0 items=["None", "Last Bit", "TermChar", "Break"] ("Serial Settings:End Mode for Writes")
          w389 = u16 0 items=["None", "Last Bit", "TermChar"] ("Serial Settings:End Mode for Reads")
          n84 = property on="Property Node" class="Instr"(reference=w381, error in=w382, "Serial Settings:End Mode for Reads"=w389, "Serial Settings:End Mode for Writes"=w388) -> (reference out=w385:refnum<visa-resource-name>, error out=w386:errorcluster, "Baud"=w380:u32)
          n85 = case shown="1, Default" w387 {
            selector: w387 -> [_ w392]
            tunnel: w386 -> [w390 w396]
            tunnel: w385 -> [w391 w393]
            tunnel: [w390 w395] -> w384
            tunnel: [w391 w394] -> w383
            tunnel: w380 -> [_ _]
            frame 0 {
            }
            frame 1, Default {
              n86 = property on="Property Node" class="Instr"(reference=w393, error in=w396, "Baud"=w392) -> (reference out=w394:refnum<visa-resource-name>, error out=w395:errorcluster)
            }
          }
        }
      }
      n87 = case "True: VXI-11 settings\nFalse: Non-VXI-11 session" shown="False" w329 {
        tunnel: w338 -> [w372 w376]
        tunnel: w337 -> [w373 w377]
        tunnel: [w361 w376] -> w336
        tunnel: [w360 w377] -> w335
        frame False {
          w374 = u8 10  # TermChar (LF)
          w375 = TRUE  # Read TermChar En
          n88 = call "session_set_one_property_boolean.vi"("Session Parameter Boolean"=type_Session_Parameter_Boolean."Add LF to Write" ("Session Parameter boolean"), "error in"=w372, "Boolean value in"=TRUE ("boolean value in"), "VISA resource name"=w373) -> ("error out"=w369:errorcluster, "VISA resource name out"=w370:refnum<visa-resource-name>)  [unwired: 5 in, 1 out]
          n89 = call "session_set_additional_flag.vi"("AdditionalFlag Bit"=type_AdditionalFlag_Bits."Send LF after Bin Block" ("AdditionalFlag bit"), "error in"=w369, "New value in"=TRUE, "VISA resource name"=w370) -> ("error out"=w367:errorcluster, "VISA resource name out"=w368:refnum<visa-resource-name>)  [unwired: 5 in, 1 out]
          n90 = property on="Property Node" class="Instr"(reference=w368, error in=w367, "Message Based Settings:Termination Character"=w374, "Message Based Settings:Termination Character Enable"=w375) -> (reference out=w359:refnum<visa-resource-name>, error out=w362:errorcluster)
          n91 = call "session_set_additional_flag.vi"("AdditionalFlag Bit"=type_AdditionalFlag_Bits."Allow Dbl & Int Bin/Ascii read" ("AdditionalFlag bit"), "error in"=w362, "New value in"=FALSE, "VISA resource name"=w359) -> ("error out"=w361:errorcluster, "VISA resource name out"=w360:refnum<visa-resource-name>)  [unwired: 5 in, 1 out]
        }
        frame True {
        }
      }
    }
    frame True {
      n92 = case "True: Simulate duplicating the session" shown="True" w422 {
        tunnel: w421 -> [w439 w441]
        tunnel: [w439 w440] -> w417
        tunnel: w420 -> [w438 w443]
        tunnel: [w438 w442] -> w418
        frame False {
        }
        frame True {
          n93 = while {
            tunnel: w443 -> [w452]
            tunnel: [w451] -> w442
            shift-right: [w446] -> w440
            shift-left: w441 -> [w450]
            stop <- w445 continue-if-true
            w447 = "(.*?)\\s*(?:\\((\\d+)\\))*$"  # Split Session and (%d)
            n94 = call "_fgv_sessions.vi"("Operation"=_type_Operation_Fgv_Session."GetSessionIx", "error in"=w452, "VISA resource name"=w450) -> ("error out"=w451:errorcluster, "Session Ix out"=w449:i32, "VISA resource name out"=w448:refnum<visa-resource-name>)  [unwired: 5 in, 1 out]
            n95 = Greater Or Equal To 0?(x=w449) -> (x >= 0?=w445:bool)
            n96 = case "True: Session already exists, add \"_(i+1)\"" shown="True" w445 {
              tunnel: w448 -> [w453 w454]
              tunnel: w447 -> [_ w462]
              tunnel: [w453 w455] -> w446
              frame False {
              }
              frame True {
                n97 = xnode "Match Regular Expression"("input string"=w454, "regular expression"=w462) -> ("submatch 1"=w458:string, "submatch 2"=w461:string)  [unwired: 4 in, 5 out]
                n98 = call "convert_string_to_int32.vi"("String in"=w461) -> ("int32 value out"=w460:i32)  [unwired: 4 in]
                n99 = Increment(x=w460) -> (x+1=w457:i32)
                n100 = Format Into String(format string="%s (%d)", w458, w457) -> (resulting string=w456:string)  [unwired: 2 in, 1 out]
                n101 = Type Cast(type=w454, x=w456) -> (*(type *) &x=w455:refnum<visa-resource-name>)
              }
            }
          }
        }
      }
      n102 = Concatenate Strings("Rohde&Schwarz," ("read buffer"), w419, ",100001,1.00" ("string")) -> (w423:string)
      n103 = Unbundle By Name(w412) -> ("Interface Type"=w411:T1)
      n104 = Search 1D Array(1D array=w410, element=w411) -> (index of element=w409:i32)  [unwired: 1 in]
      n105 = Less Than 0?(x=w409) -> (x < 0?=w408:bool)
      n106 = Bundle By Name(cluster=w412, "VXIcapable"=w408) -> (w407:T8)
      n107 = call "_fgv_sessions.vi"("Operation"=_type_Operation_Fgv_Session."Initialize", "error in"=w418, "Session User Data in (None)"=w407, "VISA resource name"=w417) -> ("error out"=w416:errorcluster, "VISA resource name out"=w415:refnum<visa-resource-name>)  [unwired: 4 in, 2 out]
      n108 = case "True: VXI-11 settings\nFalse: Non-VXI-11 session" shown="False" w408 {
        tunnel: w416 -> [w425 w436]
        tunnel: w415 -> [w426 w435]
        tunnel: [w425 w431] -> w414
        tunnel: [w426 w430] -> w413
        frame True {
        }
        frame False {
          w427 = TRUE  # Skip setting if in option string
          n109 = call "session_set_one_property_boolean.vi"("Skip setting if in Options string (F)"=w427, "Session Parameter Boolean"=type_Session_Parameter_Boolean."Add LF to Write" ("Session Parameter boolean"), "error in"=w436, "Boolean value in"=TRUE ("boolean value in"), "VISA resource name"=w435) -> ("error out"=w433:errorcluster, "VISA resource name out"=w432:refnum<visa-resource-name>)  [unwired: 4 in, 1 out]
          n110 = call "session_set_additional_flag.vi"("Skip setting if in Options string (F)"=w427, "AdditionalFlag Bit"=type_AdditionalFlag_Bits."Allow Dbl & Int Bin/Ascii read" ("AdditionalFlag bit"), "error in"=w433, "New value in"=FALSE, "VISA resource name"=w432) -> ("error out"=w431:errorcluster, "VISA resource name out"=w430:refnum<visa-resource-name>)  [unwired: 4 in, 1 out]
        }
      }
    }
  }
  "Simulation *IDN? response out" <- w55
  n111 = case "True: Set VISA Timeout to the session" shown="True" w29 {
    tunnel: w35 -> [w583 w591]
    tunnel: w34 -> [w584 w590]
    tunnel: [w583 w589] -> w13
    tunnel: [w584 w588] -> w12
    tunnel: w28 -> [_ w587]
    frame False {
    }
    frame True {
      w585 = FALSE  # Skip setting if in option string
      n112 = call "session_set_one_property_int32.vi"("Skip setting if in Options string (F)"=w585, "Session Parameter Integer"=type_Session_Parameter_int32."VISA Timeout" ("Session Parameter to set"), "error in"=w591, "Int32 value in"=w587, "VISA resource name"=w590) -> ("error out"=w589:errorcluster, "VISA resource name out"=w588:refnum<visa-resource-name>)  [unwired: 4 in, 1 out]
    }
  }
  n113 = call "session_get_data.vi"("error in"=w13, "VISA resource name"=w12) -> ("error out"=w11:errorcluster, "Session User Data out"=w9:T8, "VISA resource name out"=w10:refnum<visa-resource-name>)  [unwired: 6 in, 1 out]
  n114 = Unbundle By Name(w9) -> ("OPC Wait Mode"=w8:T10)
  n115 = call "session_set_one_property_int32.vi"("Skip setting if in Options string (F)"=w7, "Session Parameter Integer"=type_Session_Parameter_int32."OPCwaitMode" ("Session Parameter to set"), "error in"=w11, "Int32 value in"=w8, "VISA resource name"=w10) -> ("error out"=w15:errorcluster, "VISA resource name out"=w14:refnum<visa-resource-name>)  [unwired: 4 in, 1 out]
  n116 = call "rep_cap_init_all.vi"("error in"=w15, "Repeated Capabilities"="Repeated Capabilities", "VISA resource name"=w14) -> ("error out"=w63:errorcluster, "VISA resource name out"=w21:refnum<visa-resource-name>)  [unwired: 7 in]
  n117 = call "_fgv_range_tables.vi"("Range Tables (empty)"="Range Tables", "Operation"=_type_Operation_Fgv_RangeTable."Initialize", "error in"=w63, "Range Table ID in"="" ("Empty String Constant"), "VISA resource name"=w21) -> ("error out"=w77:errorcluster, "VISA resource name out"=w19:refnum<visa-resource-name>)  [unwired: 2 in, 3 out]
  n118 = call "_fgv_attributes.vi"("Attributes (empty)"="Attributes", "Operation"=_type_Operation_Fgv_Attributes."Initialize", "error in"=w77, "Attribute ID in"="" ("Empty String Constant"), "VISA resource name"=w19) -> ("error out"=w76:errorcluster, "Count Out"=w39:i32, "VISA resource name out"=w20:refnum<visa-resource-name>)  [unwired: 3 in, 1 out]
  n119 = call "_fgv_cache.vi"("Index in"=w38, "Operation"=_type_Operation_Fgv_Cache."Initialize", "error in"=w76, "Initialization Count (0)"=w39, "Value in"=w80, "VISA resource name"=w20) -> ("error out"=w73:errorcluster, "VISA resource name out"=w72:refnum<visa-resource-name>)  [unwired: 3 in, 1 out]
  n120 = disable-structure "DriverDebugging_DiagramDisabledStructure" shown="Enabled" {
    disable-tunnel: w73 -> [w597 w598]
    disable-tunnel: [w595 w598] -> w68
    disable-tunnel: w72 -> [w596 w599]
    disable-tunnel: [w594 w599] -> w67
    frame Disabled {
      # "Debug"
      n121 = call "_fgv_debug.vi"("Operation"=_type_Operation_Fgv_Debug."Reset", "error in"=w597, "Command in"="" ("Empty String Constant"), "VISA resource name"=w596) -> ("error out"=w595:errorcluster, "VISA resource name out"=w594:refnum<visa-resource-name>)  [unwired: 6 in]
    }
    frame Enabled {
      # "Release"
    }
  }
  n122 = Empty String/Path?(string/path=w64) -> (empty?=w65:bool)
  n123 = case "False: Start Logging" shown="False" w65 {
    tunnel: w68 -> [w622 w624]
    tunnel: w67 -> [w621 w625]
    tunnel: [w616 w624] -> w47
    tunnel: [w615 w625] -> w48
    tunnel: w64 -> [w623 _]
    frame False {
      w601 = TRUE  # Evaluate section error
      n124 = call "logging_set.vi"("error in"=w622, "Logging target"=w623, "VISA resource name"=w621) -> ("error out"=w620:errorcluster, "VISA resource name out"=w619:refnum<visa-resource-name>)  [unwired: 7 in]
      n125 = call "logging_start.vi"("error in"=w620, "VISA resource name"=w619) -> ("error out"=w614:errorcluster, "VISA resource name out"=w613:refnum<visa-resource-name>)  [unwired: 8 in]
      n126 = call "session_get_data.vi"("error in"=w614, "VISA resource name"=w613) -> ("error out"=w612:errorcluster, "Session Ix out"=w606:i32, "Session User Data out"=w610:T8, "VISA resource name out"=w611:refnum<visa-resource-name>)  [unwired: 6 in]
      n127 = Unbundle By Name(w610) -> ("VISA Access Mode"=w605:T9, "Interface Type"=w604:T1, "Duplicate Session"=w600:bool)
      n128 = Select(t="Duplicate", s=w600, f="Non-duplicate") -> (s? t:f=w603:string)
      n129 = Format Into String(format string="Initializing the session #%d: Access Mode %d, Interface %s, %s session", w606, w605, w604, w603) -> (resulting string=w602:string)  [unwired: 2 in, 1 out]
      n130 = call "logging_set_split.vi"("Evaluate section error (F)"=w601, "error in"=w612, "VISA resource name"=w611) -> ("error out"=w618:errorcluster, "VISA resource name out"=w617:refnum<visa-resource-name>)  [unwired: 7 in]
      n131 = call "logging_info_write.vi"("error in"=w618, "String to write"=w602, "VISA resource name"=w617) -> ("error out"=w616:errorcluster, "VISA resource name out"=w615:refnum<visa-resource-name>)  [unwired: 7 in]
    }
    frame True {
    }
  }
  n132 = call "error_filter.vi"("Error Enum in"=w57, "error in"=w47, "Clear detected code (F)"=w59, "VISA resource name"=w48) -> ("error out"=w60:errorcluster, "Code Detected"=w61:bool, "VISA resource name out"=w49:refnum<visa-resource-name>)  [unwired: 5 in]
  n133 = case "True: Resource not found" shown="True" w61 {
    tunnel: w60 -> [w627 w632]
    tunnel: [w627 w634] -> w53
    tunnel: w49 -> [w626 w628]
    tunnel: w57 -> [_ w630]
    tunnel: [w626 w629] -> w52
    frame False {
    }
    frame True {
      n134 = Format Into String(format string="The given VISA resource name \"%s\" is invalid or doesn't exist. Original VISA message: (Hex 0xBFFF0011) Insufficient location information or the device or resource is not present in the system.", w628) -> (resulting string=w631:string)  [unwired: 2 in, 1 out]
      n135 = call "error_cluster_from_error_code.vi"("error in"=w632, "Error Message (\"\")"=w631, "Error Enum in"=w630, "VISA resource name"=w628) -> ("error out"=w634:errorcluster, "VISA resource name out"=w629:refnum<visa-resource-name>)  [unwired: 6 in]
    }
  }
  n136 = call "logging_write.vi"("error in"=w53, "String to write"="viOpen", "VISA resource name"=w52) -> ("error out"=→"error out":errorcluster, "VISA resource name out"=→"VISA resource name out":refnum<visa-resource-name>)  [unwired: 7 in]
